vi "Resetting counter (SubVI).vi"(11 "Numeric":u64) -> (3 "Boolean":bool)   [LabVIEW 2025]
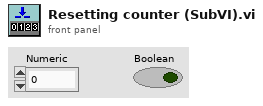
[diagram p1: front panel]
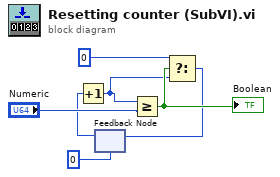
[diagram p0: block diagram]
diagram:
  n1 = feedback #1(u64 0) -> (w3:u64)
  n2 = Increment(x=w3) -> (x+1=w6:u64)
  n3 = Greater Or Equal?(x=w6, y="Numeric") -> (x >= y?=w7:bool)
  "Boolean" <- w7
  n4 = Select(t=u64 0, s=w7, f=w6) -> (s? t:f=w4:u64)
  n5 = feedback-in #1(w4) -> ()
